vi "mark time.vi"(8 "error in (no error)":errorcluster, 10 "mode":u16, 11 "part":u16) -> (0 "error out":errorcluster)   [LabVIEW 2015, in "SCANalone4x64.lvlib"]
doc: "__declspec(dllimport) void __stdcall mark_time(unsigned short part, unsigned short mode);"
uses:
  <userlib>/SCANalone4x64/SCANalone4x64.lvlib
  <userlib>/SCANalone4x64/SCANalone4x64.dll
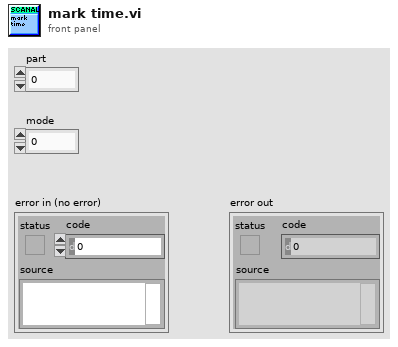
[diagram p1: front panel]
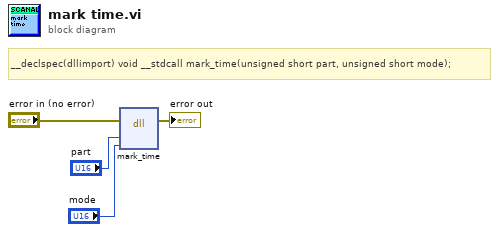
[diagram p0: block diagram]
diagram:
  # "__declspec(dllimport) void __stdcall mark_time(unsigned short part, unsigned short mode);"
  n1 = dll-call lib="C:/Program Files/National Instruments/LabVIEW 2015/user.lib/SCANalone4x64/SCANalone4x64.*" fn="mark_time"(error in="error in (no error)", "part"="part", "mode"="mode") -> (error out=→"error out":errorcluster)  [unwired: 5 in, 1 out]
